vi "Format InstanceStatusEventsSetType_LVXML.vi"(8 "error in (no error)":errorcluster, 10 "xmlData":T4, 11 "AWS_EC2 in":refnum<class "AWS_EC2.lvclass">) -> (0 "error out":errorcluster, 2 "InstanceStatusEventTypeSet":T1, 3 "AWS_EC2 out":refnum<class "AWS_EC2.lvclass">)   [LabVIEW 2014, in "AWS_EC2.lvlib" / "AWS_EC2.lvclass"]
uses:
  AWS_EC2.lvclass
  lv-xml-parser/r0/trunk/VI Source/EventType.ctl
  EC2 Datatypes/InstanceStatusEventTypeSet.ctl
  EC2 Datatypes/InstanceStatusEventType.ctl
  lv-xml-parser/r0/trunk/VI Source/LV XML Parser.lvlib
  AWS Core Lib/VI Source/AWS_Core.lvlib
  AWS_EC2.lvlib
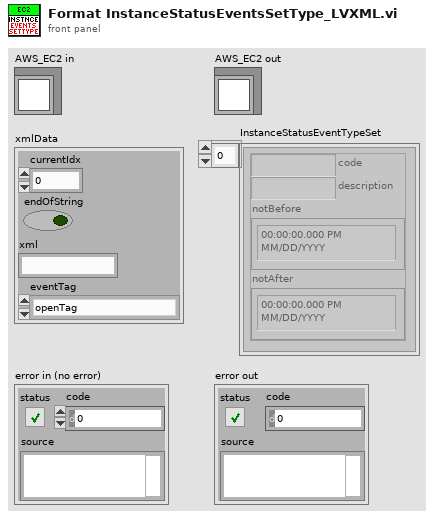
[diagram p1: front panel]
types:
  T1 = typedef "AWS_EC2.lvlib/InstanceStatusEventTypeSet.ctl" = T2[]
  T2 = typedef "AWS_EC2.lvlib/InstanceStatusEventType.ctl" = cluster{"code":string, "description":string, "notBefore":timestamp, "notAfter":timestamp}
  T3 = typedef "LV XML Parser.lvlib/EventType.ctl" = enum16{"openTag", "endOpenTag", "closeTag", "comment", "endComment", "endOfFile", "attribute", "startXml"}
  T4 = cluster{"currentIdx":i32, "endOfString":bool, "xml":string, "eventTag":T3}
  T5 = cluster{"namespaceUri":string, "localName":string}
  T6 = cluster{"Attributes":cluster{"localName":string, "namespaceUri":string, "value":string}[], "localName":string, "namespaceUri":string, "valueXmlData":cluster{"currentIdx":i32, "endOfString":bool, "xml":string, "eventTag":T3}}[]
  T7 = cluster{"Attributes":cluster{"localName":string, "namespaceUri":string, "value":string}[], "localName":string, "namespaceUri":string, "valueXmlData":cluster{"currentIdx":i32, "endOfString":bool, "xml":string, "eventTag":T3}}
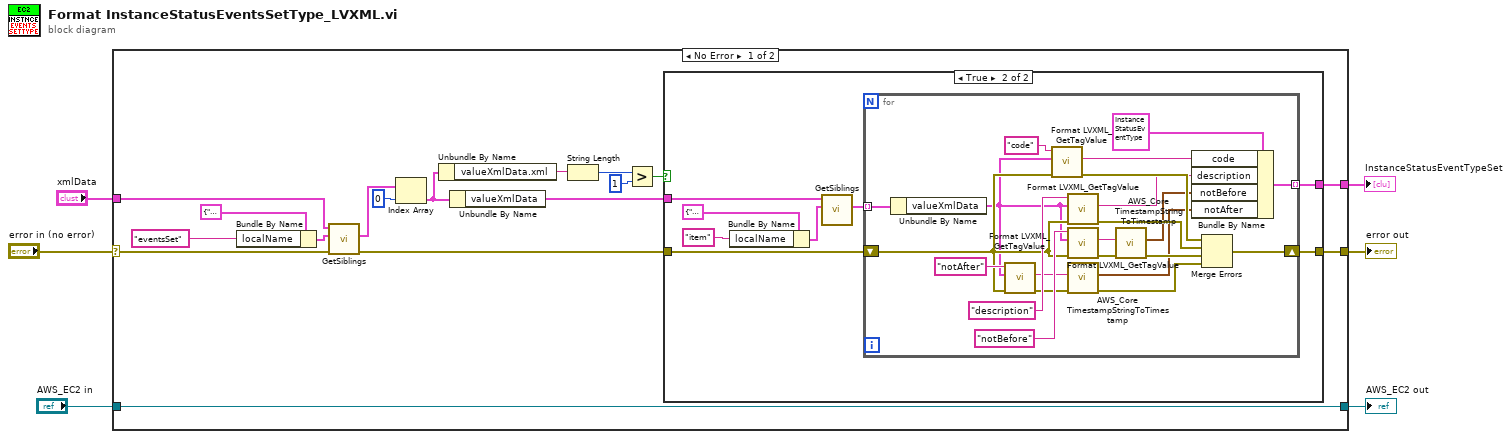
[diagram p0: block diagram]
diagram:
  n1 = case shown="No Error" "error in (no error)" {
    selector: "error in (no error)" -> [w14 w56]
    tunnel: [w17 w56] -> w4
    tunnel: [w23 w55] -> w5
    tunnel: "AWS_EC2 in" -> [w23 w55]
    tunnel: "xmlData" -> [w15 _]
    tunnel: [w11 _] -> w1
    frame No Error {
      n2 = Bundle By Name(cluster=T5 {"namespaceUri"="", "localName"=""} ("limitToTag"), "localName"="eventsSet" ("Tag name")) -> (w20:T5)
      n3 = call "GetSiblings.vi"("error in (no error)"=w14, "limitToTag"=w20, "xmlData"=w15) -> ("error out"=w16:errorcluster, "Siblings"=w19:T6)  [unwired: 7 in]
      n4 = Index Array(array=w19, index=0) -> (element=w13:T7)
      n5 = Unbundle By Name(w13) -> ("valueXmlData.xml"=w8:string)
      n6 = Unbundle By Name(w13) -> ("valueXmlData"=w12:T4)
      n7 = String Length(string=w8) -> (length=w9:i32)
      n8 = Greater?(x=w9, y=1) -> (0:w7:bool)
      n9 = case shown="True" w7 {
        tunnel: [w24 w32] -> w17
        tunnel: w16 -> [w24 w31]
        tunnel: w12 -> [_ w27]
        tunnel: [_ w25] -> w11
        frame False {
        }
        frame True {
          n10 = Bundle By Name(cluster=T5 {"namespaceUri"="", "localName"=""} ("limitToTag"), "localName"="item" ("Tag name")) -> (w30:T5)
          n11 = call "GetSiblings.vi"("limitToTag"=w30, "xmlData"=w27) -> ("Siblings"=w26:T6)  [unwired: 8 in, 1 out]
          n12 = for {
            tunnel: w26 -> [w36] mode=indexing
            tunnel: [w34] -> w25 mode=indexing
            shift-right: [w54] -> w32
            shift-left: w31 -> [w44]
            n13 = Unbundle By Name(w36) -> ("valueXmlData"=w35:T4)
            n14 = call "Format LVXML_GetTagValue.vi"("error in (no error)"=w44, "xmlDataIn"=w35, "Tag name"="notAfter") -> ("error out"=w41:errorcluster, "Value"=w40:string)  [unwired: 6 in, 1 out]
            n15 = call "Format LVXML_GetTagValue.vi"("error in (no error)"=w44, "xmlDataIn"=w35, "Tag name"="code") -> ("error out"=w53:errorcluster, "Value"=w43:string)  [unwired: 6 in, 1 out]
            n16 = call "Format LVXML_GetTagValue.vi"("error in (no error)"=w44, "xmlDataIn"=w35, "Tag name"="description") -> ("error out"=w50:errorcluster, "Value"=w42:string)  [unwired: 6 in, 1 out]
            n17 = call "Format LVXML_GetTagValue.vi"("error in (no error)"=w44, "xmlDataIn"=w35, "Tag name"="notBefore") -> ("error out"=w47:errorcluster, "Value"=w48:string)  [unwired: 6 in, 1 out]
            n18 = call "AWS_Core TimestampStringToTimestamp.vi"("error in"=w41, "AWS Timestamp String"=w40) -> ("error out"=w39:errorcluster, "Time Stamp Control"=w38:timestamp)  [unwired: 8 in]
            n19 = call "AWS_Core TimestampStringToTimestamp.vi"("error in"=w47, "AWS Timestamp String"=w48) -> ("error out"=w46:errorcluster, "Time Stamp Control"=w37:timestamp)  [unwired: 8 in]
            n20 = Bundle By Name(cluster=T2 {"code"="", "description"="", "notBefore"=timestamp(0 s since 1904-01-01), "notAfter"=timestamp(0 s since 1904-01-01)} ("InstancesStatusEventType"), "code"=w43, "description"=w42, "notBefore"=w37, "notAfter"=w38) -> (w34:T2)
            n21 = Merge Errors(w53, w50, w46, w39) -> (w54:errorcluster)
          }
        }
      }
    }
    frame Error {
    }
  }
  "AWS_EC2 out" <- w5
  "error out" <- w4
  "InstanceStatusEventTypeSet" <- w1
